vi "Page_Source_Settings_UpdateDisplay_DefSaveLevel.vi"(8 "error in (no error)":errorcluster, 11 "AB_Targetfile in":refnum<class "AB_Targetfile.lvclass">) -> (0 "error out":errorcluster, 2 "defaultSaveLevel":u32, 3 "AB_Targetfile out":refnum<class "AB_Targetfile.lvclass">)   [LabVIEW 2020, in "AB_Targetfile.lvclass"]
uses:
  <vilib>/AppBuilder/AB_Classes/TargetFile/AB_Targetfile.lvclass
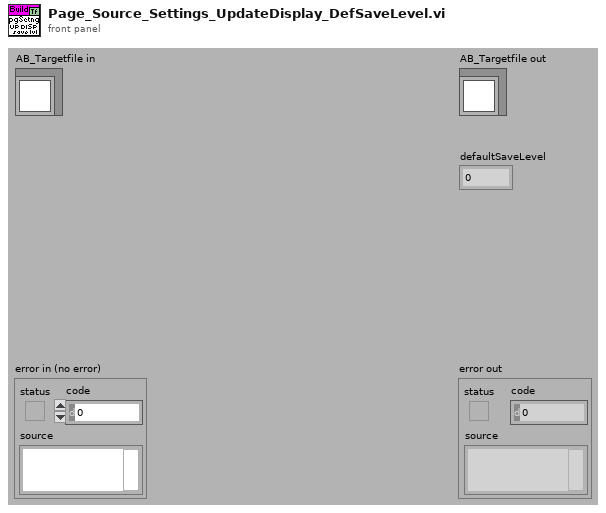
[diagram p1: front panel]
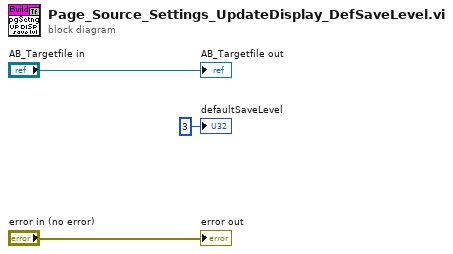
[diagram p0: block diagram]
diagram:
  "error out" <- "error in (no error)"
  "AB_Targetfile out" <- "AB_Targetfile in"
  "defaultSaveLevel" <- u32 3 ("defaultSaveLevel")
